vi "readModeXML.vi"(8 "error in (no error)":errorcluster, 10 "NativeXML in":refnum<class "NativeXML.lvclass">, 11 "PixelflySettings in":refnum<class "PixelflySettings.lvclass">) -> (0 "error out":errorcluster, 2 "NativeXML out":refnum<class "NativeXML.lvclass">, 3 "PixelflySettings out":refnum<class "PixelflySettings.lvclass">)   [LabVIEW 2011, in "Tools.lvlib" / "Settings.lvlib" / "PixelflySettings.lvclass"]
uses:
  PixelflySettings.lvclass
  NativeXML/NativeXML.lvclass
  PixelflySettings.lvclass/PixelflySettings.ctl
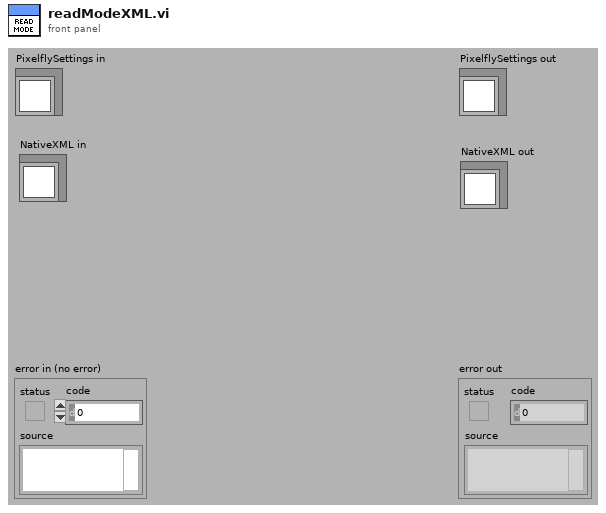
[diagram p1: front panel]
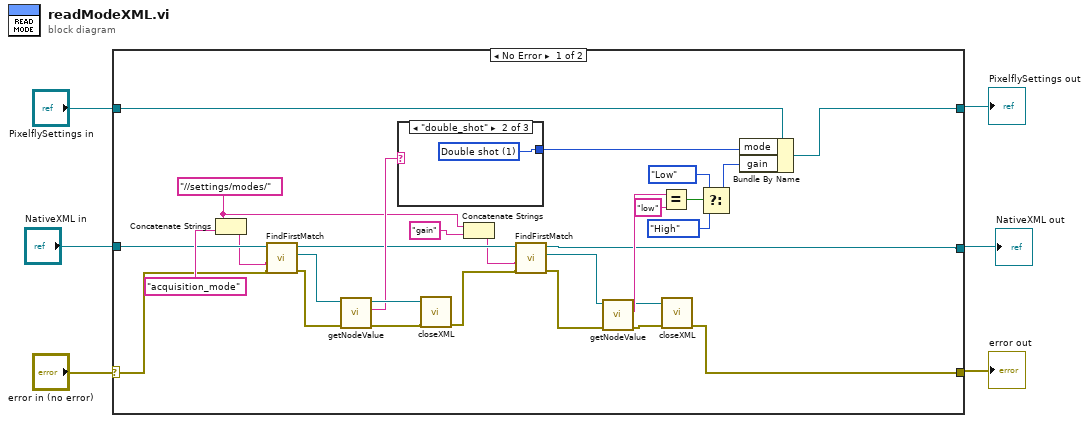
[diagram p0: block diagram]
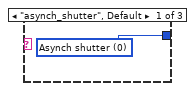
[diagram p2: hidden frame]
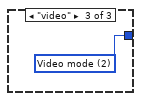
[diagram p3: hidden frame]
diagram:
  n1 = case shown="No Error" "error in (no error)" {
    selector: "error in (no error)" -> [w14 w41]
    tunnel: [w25 w41] -> w5
    tunnel: [w31 w40] -> w3
    tunnel: "PixelflySettings in" -> [w32 w40]
    tunnel: "NativeXML in" -> [w17 w39]
    tunnel: [w11 w39] -> w1
    frame No Error {
      w19 = "//settings/modes/" ("searchElementIn")
      n2 = Concatenate Strings(w19, "acquisition_mode") -> (w13:string)
      n3 = call "FindFirstMatch.vi"("error in (no error)"=w14, "xPath"=w13, "NativeXML in"=w17) -> ("error out"=w15:errorcluster, "NativeXML match"=w16:refnum<class "NativeXML.lvclass">, "NativeXML out"=w12:refnum<class "NativeXML.lvclass">)  [unwired: 6 in]
      n4 = call "getNodeValue.vi"("error in (no error)"=w15, "NativeXML in"=w16) -> ("error out"=w23:errorcluster, "Value"=w22:string, "NativeXML out"=w24:refnum<class "NativeXML.lvclass">)  [unwired: 7 in]
      n5 = case shown="\"double_shot\"" w22 {
        tunnel: [w36 w37 w38] -> w21
        frame "asynch_shutter", Default {
          w36 = u16 0 items=["Asynch shutter", "Double shot", "Video mode", "Auto exposure"] ("Exposure mode")
        }
        frame "double_shot" {
          w37 = u16 1 items=["Asynch shutter", "Double shot", "Video mode", "Auto exposure"] ("Exposure mode")
        }
        frame "video" {
          w38 = u16 2 items=["Asynch shutter", "Double shot", "Video mode", "Auto exposure"] ("Exposure mode")
        }
      }
      n6 = call "closeXML.vi"("error in (no error)"=w23, "NativeXML in"=w24) -> ("error out"=w7:errorcluster)  [unwired: 9 in]
      n7 = Concatenate Strings(w19, "gain" ("searchElementName")) -> (w8:string)
      n8 = call "FindFirstMatch.vi"("error in (no error)"=w7, "xPath"=w8, "NativeXML in"=w12) -> ("error out"=w10:errorcluster, "NativeXML match"=w9:refnum<class "NativeXML.lvclass">, "NativeXML out"=w11:refnum<class "NativeXML.lvclass">)  [unwired: 6 in]
      n9 = call "getNodeValue.vi"("error in (no error)"=w10, "NativeXML in"=w9) -> ("error out"=w26:errorcluster, "Value"=w34:string, "NativeXML out"=w27:refnum<class "NativeXML.lvclass">)  [unwired: 7 in]
      n10 = Equal?(x=w34, y="low" ("searchElementName")) -> (x = y?=w35:bool)
      n11 = call "closeXML.vi"("error in (no error)"=w26, "NativeXML in"=w27) -> ("error out"=w25:errorcluster)  [unwired: 9 in]
      n12 = Select(t=enum16{"Low", "High"}."Low" ("gain"), s=w35, f=enum16{"Low", "High"}."High" ("gain")) -> (s? t:f=w30:enum16{"Low", "High"})
      n13 = Bundle By Name(cluster=w32, "mode"=w21, "gain"=w30) -> (w31:refnum<class "PixelflySettings.lvclass">)
    }
    frame Error {
    }
  }
  "error out" <- w5
  "PixelflySettings out" <- w3
  "NativeXML out" <- w1
